vi "S4GUI.vi"(7 "Tab ObsEng":enum32{"Obs", "CCD modes", "Guider", "Eng"}(tab)) -> ()   [LabVIEW 2018] (continued)
                    n880 = Not(x=w1537) -> (.not. x?=w1558:bool)
                    n881 = Not(x=w1536) -> (.not. x?=w1557:bool)
                    n882 = Not(x=w1535) -> (.not. x?=w1559:bool)
                    n883 = property on="Acquisition Mode 2" class="Ring (strict)"("Blinking"=w1553) -> ()  [unwired: 2 in, 2 out]
                    n884 = property on="Readout Rate 2" class="Ring (strict)"("Blinking"=w1556) -> ()  [unwired: 2 in, 2 out]
                    n885 = property on="Vertical Shift Speed 2" class="Ring (strict)"("Blinking"=w1554) -> ()  [unwired: 2 in, 2 out]
                    n886 = property on="CCD EM Mode 2" class="Ring (strict)"("Blinking"=w1555) -> ()  [unwired: 2 in, 2 out]
                    n887 = property on="Trigger Mode 2" class="Ring (strict)"("Blinking"=w1558) -> ()  [unwired: 2 in, 2 out]
                    n888 = property on="Read Mode 2" class="Ring (strict)"("Blinking"=w1557) -> ()  [unwired: 2 in, 2 out]
                    n889 = property on="Pre-amplification Gain 2" class="Ring (strict)"("Blinking"=w1559) -> ()  [unwired: 2 in, 2 out]
                  }
                }
                n890 = local read "Cameras Cluster"() -> (w1523:T7)
                n891 = Bundle By Name(cluster=w1523, "Current Configuration.Image Initial Line 2"=w1486, "Current Configuration.Image Initial Column 2"=w1484, "Current Configuration.Image Final Line 2"=w1487, "Current Configuration.Image FInal Column 2"=w1485, "Current Configuration.Vertical Binning 2"=w1490, "Current Configuration.Horizontal Binning 2"=w1521, "Current Configuration.Pre-amplification Gain 2"=w1489, "Current Configuration.CCD EM Gain 2"=w1488, "Current Configuration.Readout Rate 2"=w1483, "Current Configuration.Shutter Openning Time 2"=w1520, "Current Configuration.Shutter Closing Time 2"=w1519, "Current Configuration.Vertical Shift Speed 2"=w1518, "Current Configuration.Read Mode 2"=w1517, "Current Configuration.Vertical Clock Voltage 2"=w1516, "Current Configuration.A/D Channel 2"=w1515, "Current Configuration.Shutter Mode 2"=w1512, "Current Configuration.Shutter TTL 2"=w1513, "Current Configuration.Trigger Mode 2"=w1491, "Current Configuration.Frame Transfer 2"=w1492, "Current Configuration.Acquisition Mode 2"=w1514, "Current Configuration.CCD EM Mode 2"=w1482) -> (w1522:T7)
                n892 = local write "PA2"(w1477) -> ()
                n893 = local write "B2"(w1476) -> ()
                n894 = local write "EA2"(w1478) -> ()
                n895 = local write "SI2"(w1473) -> ()
                n896 = local write "RO2"(w1474) -> ()
                n897 = local write "G2"(w1475) -> ()
                n898 = local write "Cameras Cluster"(w1522) -> ()
                n899 = Compound Arithmetic op=AND(w1497, w1496, w1495, w1494, w1470, w1469, w1493, w1504, w1503, w1502, w1501, w1500, w1499, w1498, w1511, w1510, w1509, w1508, w1507, w1506, w1505) -> (w1468:bool)
                "CCD checked 2" <- w1468
                n900 = disable-structure shown="Disabled" {
                  disable-tunnel: w1468 -> [w1525 _]
                  frame Disabled {
                    n901 = Select(t=u32 1244955, s=w1525, f=u32 16718848) -> (s? t:f=w1528:u32)
                    n902 = property on="CCD checked 2" class="Bool (strict)"("Caption.BG Color"=w1528) -> ()  [unwired: 2 in, 2 out]
                  }
                  frame Enabled {
                  }
                }
                n903 = property on="Acquisition Mode 2" class="Ring (strict)"("DisabledEnum"=w1471) -> ()  [unwired: 2 in, 2 out]
                n904 = property on="Readout Rate 2" class="Ring (strict)"("DisabledEnum"=w1471) -> ()  [unwired: 2 in, 2 out]
                n905 = property on="Vertical Shift Speed 2" class="Ring (strict)"("DisabledEnum"=w1471) -> ()  [unwired: 2 in, 2 out]
                n906 = property on="CCD EM Mode 2" class="Ring (strict)"("DisabledEnum"=w1471) -> ()  [unwired: 2 in, 2 out]
                n907 = property on="Shutter Openning Time 2" class="DigNum (strict)"("DisabledEnum"=w1471) -> ()  [unwired: 2 in, 2 out]
                n908 = property on="Shutter Closing Time 2" class="DigNum (strict)"("DisabledEnum"=w1471) -> ()  [unwired: 2 in, 2 out]
                n909 = property on="Vertical Binning 2" class="DigNum (strict)"("DisabledEnum"=w1471) -> ()  [unwired: 2 in, 2 out]
                n910 = property on="Horizontal Binning 2" class="DigNum (strict)"("DisabledEnum"=w1471) -> ()  [unwired: 2 in, 2 out]
                n911 = property on="Trigger Mode 2" class="Ring (strict)"("DisabledEnum"=w1471) -> ()  [unwired: 2 in, 2 out]
                n912 = property on="Read Mode 2" class="Ring (strict)"("DisabledEnum"=w1471) -> ()  [unwired: 2 in, 2 out]
                n913 = property on="Pre-amplification Gain 2" class="Ring (strict)"("DisabledEnum"=w1471) -> ()  [unwired: 2 in, 2 out]
                n914 = property on="CCD EM Gain 2" class="DigNum (strict)"("DisabledEnum"=w1471) -> ()  [unwired: 2 in, 2 out]
                n915 = property on="Shutter Mode 2" class="Ring (strict)"("DisabledEnum"=w1471) -> ()  [unwired: 2 in, 2 out]
                n916 = property on="Shutter TTL 2" class="Ring (strict)"("DisabledEnum"=w1471) -> ()  [unwired: 2 in, 2 out]
                n917 = property on="Image FInal Column 2" class="DigNum (strict)"("DisabledEnum"=w1471) -> ()  [unwired: 2 in, 2 out]
                n918 = property on="Frame Transfer 2" class="Bool (strict)"("DisabledEnum"=w1471) -> ()  [unwired: 2 in, 2 out]
                n919 = property on="Vertical Clock Voltage 2" class="Ring (strict)"("DisabledEnum"=w1471) -> ()  [unwired: 2 in, 2 out]
                n920 = property on="A/D Channel 2" class="DigNum (strict)"("DisabledEnum"=w1471) -> ()  [unwired: 2 in, 2 out]
                n921 = property on="Image Initial Line 2" class="DigNum (strict)"("DisabledEnum"=w1471) -> ()  [unwired: 2 in, 2 out]
                n922 = property on="Image Initial Column 2" class="DigNum (strict)"("DisabledEnum"=w1471) -> ()  [unwired: 2 in, 2 out]
                n923 = property on="Image Final Line 2" class="DigNum (strict)"("DisabledEnum"=w1471) -> ()  [unwired: 2 in, 2 out]
              }
              frame #17 {
                # "Carrega coluna do Channel 3"
                # "Aba:  Eng->Camera"
                n924 = Unbundle By Name(w1687) -> ("ChannelC_CCD"=w1657:T29, "CHC_Checked Params"=w1672:T14, "ChannelC_Status.connection"=w1650:bool)
                n925 = Unbundle By Name(w1672) -> ("ACQUISITION_MODE"=w1639:bool, "TRIGGER_MODE"=w1638:bool, "READ_MODE"=w1637:bool, "PREAMP"=w1636:bool, "READOUT_RATE"=w1635:bool, "VERTICAL_SHIFT_SPEED"=w1634:bool, "EM_MODE"=w1633:bool, "EM_GAIN"=w1670:bool, "SHUTTER_MODE"=w1669:bool, "SHUTTER_TTL"=w1668:bool, "SHUTTER_OPENING_TIME"=w1667:bool, "SHUTTER_CLOSING_TIME"=w1649:bool, "VBIN"=w1641:bool, "HBIN"=w1640:bool, "INITIAL_LINE"=w1648:bool, "INITIAL_COLUMN"=w1647:bool, "FINAL_LINE"=w1646:bool, "FINAL_COLUMN"=w1645:bool, "FRAME_TRANSFER"=w1644:bool, "VERTICAL_CLOCK_VOLTAGE"=w1643:bool, "AD_CHANNEL"=w1642:bool)
                n926 = case shown="True" w1650 {
                  tunnel: w1657 -> [_ w1740]
                  tunnel: [w1733 w1739] -> w1656
                  tunnel: [w1733 w1738] -> w1655
                  tunnel: [w1733 w1737] -> w1654
                  tunnel: [w1733 w1736] -> w1653
                  tunnel: [w1733 w1735] -> w1652
                  tunnel: [w1733 w1734] -> w1651
                  frame False {
                    w1733 = ""
                  }
                  frame True {
                    n927 = stacked-sequence "Atualizacao dos indicadores inferiores do CANAL C da tela principal" {
                      tunnel: w1740 -> [w1755 w1758 w1763 w1772 w1775 w1779]
                      tunnel: [w1741 _ _ _ _ _] -> w1739
                      tunnel: [_ w1756 _ _ _ _] -> w1738
                      tunnel: [_ _ w1761 _ _ _] -> w1737
                      tunnel: [_ _ _ w1766 _ _] -> w1736
                      tunnel: [_ _ _ _ w1773 _] -> w1735
                      tunnel: [_ _ _ _ _ w1776] -> w1734
                      frame #0 {
                        # "SubImage"
                        n928 = Unbundle By Name(w1755) -> ("INITIAL_LINE"=w1753:u16, "FINAL_LINE"=w1752:u16, "INITIAL_COLUMN"=w1751:u16, "FINAL_COLUMN"=w1750:u16)
                        n929 = Number To Decimal String(number=w1753) -> (decimal integer string=w1749:string)  [unwired: 1 in]
                        n930 = Number To Decimal String(number=w1752) -> (decimal integer string=w1747:string)  [unwired: 1 in]
                        n931 = Number To Decimal String(number=w1751) -> (decimal integer string=w1745:string)  [unwired: 1 in]
                        n932 = Number To Decimal String(number=w1750) -> (decimal integer string=w1743:string)  [unwired: 1 in]
                        n933 = Concatenate Strings("[", w1749, ":", w1747, ",", w1745, ":", w1743, "]") -> (w1741:string)
                      }
                      frame #1 {
                        # "Em Active"
                        n934 = Unbundle By Name(w1758) -> ("EM_MODE"=w1757:u8)
                        n935 = case shown="0, Default" w1757 {
                          tunnel: ["Electron M." ("EmActive1") "Convent." ("EmActive1")] -> w1756
                          frame 0, Default {
                          }
                          frame 1 {
                          }
                        }
                      }
                      frame #2 {
                        # "Pre Amp"
                        n936 = Unbundle By Name(w1763) -> ("PREAMP"=w1762:u8)
                        n937 = case shown="1" w1762 {
                          tunnel: ["Gain 1" ("EmActive1") "Gain 2" ("EmActive1")] -> w1761
                          frame 0, Default {
                          }
                          frame 1 {
                          }
                        }
                      }
                      frame #3 {
                        # "Binning"
                        n938 = Unbundle By Name(w1772) -> ("VBIN"=w1771:u16, "HBIN"=w1770:u16)
                        n939 = Number To Decimal String(number=w1770) -> (decimal integer string=w1767:string)  [unwired: 1 in]
                        n940 = Number To Decimal String(number=w1771) -> (decimal integer string=w1769:string)  [unwired: 1 in]
                        n941 = Concatenate Strings(w1769, "x", w1767) -> (w1766:string)
                      }
                      frame #4 {
                        # "Gain"
                        n942 = Unbundle By Name(w1775) -> ("EM_GAIN"=w1774:u16)
                        n943 = Number To Decimal String(number=w1774) -> (decimal integer string=w1773:string)  [unwired: 1 in]
                      }
                      frame #5 {
                        # "Readout"
                        n944 = Unbundle By Name(w1779) -> ("EM_MODE"=w1778:u8, "READOUT_RATE"=w1777:u8)
                        n945 = case shown="0, Default" w1778 {
                          tunnel: w1777 -> [w1781 w1787]
                          tunnel: [w1780 w1786] -> w1776
                          frame 0, Default {
                            n946 = case shown="3" w1781 {
                              tunnel: ["30 MHz" ("EmActive1") "20 MHz" ("EmActive1") "10 MHz" ("EmActive1") "1 MHz" ("EmActive1")] -> w1780
                              frame 0, Default {
                              }
                              frame 1 {
                              }
                              frame 2 {
                              }
                              frame 3 {
                              }
                            }
                          }
                          frame 1 {
                            n947 = case shown="1" w1787 {
                              tunnel: ["1 MHz" ("EmActive1") "0.1 MHz" ("EmActive1")] -> w1786
                              frame 0, Default {
                              }
                              frame 1 {
                              }
                            }
                          }
                        }
                      }
                    }
                  }
                }
                n948 = Unbundle By Name(w1657) -> ("INITIAL_LINE"=w1662:u16, "INITIAL_COLUMN"=w1660:u16, "FINAL_LINE"=w1663:u16, "FINAL_COLUMN"=w1661:u16, "VBIN"=w1666:u16, "HBIN"=w1684:u16, "PREAMP"=w1665:u8, "EM_GAIN"=w1664:u16, "READOUT_RATE"=w1659:u8, "SHUTTER_OPENNING_TIME"=w1683:u16, "SHUTTER_CLOSING_TIME"=w1682:u16, "VERTICAL_SHIFT_SPEED"=w1681:u8, "READ_MODE"=w1680:u8, "VERTICAL_CLOCK_VOLTAGE"=w1679:u8, "AD_CHANNEL"=w1678:u32, "SHUTTER_MODE"=w1673:u8, "SHUTTER_TTL"=w1674:u8, "TRIGGER_MODE"=w1675:u8, "FRAME_TRANSFER"=w1676:bool, "ACQUISITION_MODE"=w1677:u8, "EM_MODE"=w1658:u8)
                n949 = local read "CH3 on"() -> (w1632:bool)
                n950 = case shown="True" w1632 {
                  tunnel: w1670 -> [_ w1713]
                  tunnel: w1669 -> [_ w1712]
                  tunnel: w1668 -> [_ w1710]
                  tunnel: w1667 -> [_ w1709]
                  tunnel: w1649 -> [_ w1708]
                  tunnel: w1648 -> [_ w1707]
                  tunnel: w1647 -> [_ w1706]
                  tunnel: w1646 -> [_ w1705]
                  tunnel: w1645 -> [_ w1704]
                  tunnel: w1644 -> [_ w1703]
                  tunnel: w1643 -> [_ w1702]
                  tunnel: w1642 -> [_ w1701]
                  tunnel: w1641 -> [_ w1700]
                  tunnel: w1640 -> [_ w1699]
                  tunnel: w1639 -> [_ w1698]
                  tunnel: w1638 -> [_ w1697]
                  tunnel: w1637 -> [_ w1696]
                  tunnel: w1636 -> [_ w1695]
                  tunnel: w1635 -> [_ w1694]
                  tunnel: w1634 -> [_ w1693]
                  tunnel: w1633 -> [_ w1692]
                  tunnel: [T12."Disabled and Grayed Out" ("Disabled") T12."Enabled" ("Disabled")] -> w1631
                  frame False {
                    w1688 = FALSE
                    n951 = property on="Image Initial Line 3" class="DigNum (strict)"("Blinking"=w1688) -> ()  [unwired: 2 in, 2 out]
                    n952 = property on="Image Initial Column 3" class="DigNum (strict)"("Blinking"=w1688) -> ()  [unwired: 2 in, 2 out]
                    n953 = property on="Image Final Line 3" class="DigNum (strict)"("Blinking"=w1688) -> ()  [unwired: 2 in, 2 out]
                    n954 = property on="Image FInal Column 3" class="DigNum (strict)"("Blinking"=w1688) -> ()  [unwired: 2 in, 2 out]
                    n955 = property on="Frame Transfer 3" class="Bool (strict)"("Blinking"=w1688) -> ()  [unwired: 2 in, 2 out]
                    n956 = property on="Vertical Clock Voltage 3" class="Ring (strict)"("Blinking"=w1688) -> ()  [unwired: 2 in, 2 out]
                    n957 = property on="A/D Channel 3" class="DigNum (strict)"("Blinking"=w1688) -> ()  [unwired: 2 in, 2 out]
                    n958 = property on="CCD EM Gain 3" class="DigNum (strict)"("Blinking"=w1688) -> ()  [unwired: 2 in, 2 out]
                    n959 = property on="Shutter Mode 3" class="Ring (strict)"("Blinking"=w1688) -> ()  [unwired: 2 in, 2 out]
                    n960 = property on="Shutter TTL 3" class="Ring (strict)"("Blinking"=w1688) -> ()  [unwired: 2 in, 2 out]
                    n961 = property on="Shutter Openning Time 3" class="DigNum (strict)"("Blinking"=w1688) -> ()  [unwired: 2 in, 2 out]
                    n962 = property on="Shutter Closing Time 3" class="DigNum (strict)"("Blinking"=w1688) -> ()  [unwired: 2 in, 2 out]
                    n963 = property on="Vertical Binning 3" class="DigNum (strict)"("Blinking"=w1688) -> ()  [unwired: 2 in, 2 out]
                    n964 = property on="Horizontal Binning 3" class="DigNum (strict)"("Blinking"=w1688) -> ()  [unwired: 2 in, 2 out]
                    n965 = property on="Acquisition Mode 3" class="Ring (strict)"("Blinking"=w1688) -> ()  [unwired: 2 in, 2 out]
                    n966 = property on="Vertical Shift Speed 3" class="Ring (strict)"("Blinking"=w1688) -> ()  [unwired: 2 in, 2 out]
                    n967 = property on="Trigger Mode 3" class="Ring (strict)"("Blinking"=w1688) -> ()  [unwired: 2 in, 2 out]
                    n968 = property on="Read Mode 3" class="Ring (strict)"("Blinking"=w1688) -> ()  [unwired: 2 in, 2 out]
                    n969 = property on="Readout Rate 3" class="Ring (strict)"("Blinking"=w1688) -> ()  [unwired: 2 in, 2 out]
                    n970 = property on="CCD EM Mode 3" class="Ring (strict)"("Blinking"=w1688) -> ()  [unwired: 2 in, 2 out]
                    n971 = property on="Pre-amplification Gain 3" class="Ring (strict)"("Blinking"=w1688) -> ()  [unwired: 2 in, 2 out]
                  }
                  frame True {
                    n972 = Not(x=w1707) -> (.not. x?=w1690:bool)
                    n973 = Not(x=w1706) -> (.not. x?=w1731:bool)
                    n974 = Not(x=w1705) -> (.not. x?=w1732:bool)
                    n975 = Not(x=w1704) -> (.not. x?=w1730:bool)
                    n976 = Not(x=w1703) -> (.not. x?=w1728:bool)
                    n977 = Not(x=w1702) -> (.not. x?=w1729:bool)
                    n978 = Not(x=w1701) -> (.not. x?=w1727:bool)
                    n979 = property on="Image FInal Column 3" class="DigNum (strict)"("Blinking"=w1730) -> ()  [unwired: 2 in, 2 out]
                    n980 = property on="Frame Transfer 3" class="Bool (strict)"("Blinking"=w1728) -> ()  [unwired: 2 in, 2 out]
                    n981 = property on="Vertical Clock Voltage 3" class="Ring (strict)"("Blinking"=w1729) -> ()  [unwired: 2 in, 2 out]
                    n982 = property on="Image Initial Line 3" class="DigNum (strict)"("Blinking"=w1690) -> ()  [unwired: 2 in, 2 out]
                    n983 = property on="Image Initial Column 3" class="DigNum (strict)"("Blinking"=w1731) -> ()  [unwired: 2 in, 2 out]
                    n984 = property on="Image Final Line 3" class="DigNum (strict)"("Blinking"=w1732) -> ()  [unwired: 2 in, 2 out]
                    n985 = property on="A/D Channel 3" class="DigNum (strict)"("Blinking"=w1727) -> ()  [unwired: 2 in, 2 out]
                    n986 = Not(x=w1709) -> (.not. x?=w1723:bool)
                    n987 = Not(x=w1708) -> (.not. x?=w1725:bool)
                    n988 = Not(x=w1700) -> (.not. x?=w1724:bool)
                    n989 = Not(x=w1699) -> (.not. x?=w1726:bool)
                    n990 = Not(x=w1713) -> (.not. x?=w1722:bool)
                    n991 = Not(x=w1712) -> (.not. x?=w1711:bool)
                    n992 = Not(x=w1710) -> (.not. x?=w1721:bool)
                    n993 = property on="Shutter Openning Time 3" class="DigNum (strict)"("Blinking"=w1723) -> ()  [unwired: 2 in, 2 out]
                    n994 = property on="Shutter Closing Time 3" class="DigNum (strict)"("Blinking"=w1725) -> ()  [unwired: 2 in, 2 out]
                    n995 = property on="Vertical Binning 3" class="DigNum (strict)"("Blinking"=w1724) -> ()  [unwired: 2 in, 2 out]
                    n996 = property on="Horizontal Binning 3" class="DigNum (strict)"("Blinking"=w1726) -> ()  [unwired: 2 in, 2 out]
                    n997 = property on="CCD EM Gain 3" class="DigNum (strict)"("Blinking"=w1722) -> ()  [unwired: 2 in, 2 out]
                    n998 = property on="Shutter Mode 3" class="Ring (strict)"("Blinking"=w1711) -> ()  [unwired: 2 in, 2 out]
                    n999 = property on="Shutter TTL 3" class="Ring (strict)"("Blinking"=w1721) -> ()  [unwired: 2 in, 2 out]
                    n1000 = Not(x=w1698) -> (.not. x?=w1714:bool)
                    n1001 = Not(x=w1694) -> (.not. x?=w1717:bool)
                    n1002 = Not(x=w1693) -> (.not. x?=w1715:bool)
                    n1003 = Not(x=w1692) -> (.not. x?=w1716:bool)
                    n1004 = Not(x=w1697) -> (.not. x?=w1719:bool)
                    n1005 = Not(x=w1696) -> (.not. x?=w1718:bool)
                    n1006 = Not(x=w1695) -> (.not. x?=w1720:bool)
                    n1007 = property on="Acquisition Mode 3" class="Ring (strict)"("Blinking"=w1714) -> ()  [unwired: 2 in, 2 out]
                    n1008 = property on="Readout Rate 3" class="Ring (strict)"("Blinking"=w1717) -> ()  [unwired: 2 in, 2 out]
                    n1009 = property on="Vertical Shift Speed 3" class="Ring (strict)"("Blinking"=w1715) -> ()  [unwired: 2 in, 2 out]
                    n1010 = property on="CCD EM Mode 3" class="Ring (strict)"("Blinking"=w1716) -> ()  [unwired: 2 in, 2 out]
                    n1011 = property on="Trigger Mode 3" class="Ring (strict)"("Blinking"=w1719) -> ()  [unwired: 2 in, 2 out]
                    n1012 = property on="Read Mode 3" class="Ring (strict)"("Blinking"=w1718) -> ()  [unwired: 2 in, 2 out]
                    n1013 = property on="Pre-amplification Gain 3" class="Ring (strict)"("Blinking"=w1720) -> ()  [unwired: 2 in, 2 out]
                  }
                }
                n1014 = local write "RO3"(w1651) -> ()
                n1015 = local write "B3"(w1653) -> ()
                n1016 = local write "PA3"(w1654) -> ()
                n1017 = local write "EA3"(w1655) -> ()
                n1018 = local write "G3"(w1652) -> ()
                n1019 = local write "SI3"(w1656) -> ()
                n1020 = local read "Cameras Cluster"() -> (w1686:T7)
                n1021 = Bundle By Name(cluster=w1686, "Current Configuration.Image Initial Line 3"=w1662, "Current Configuration.Image Initial Column 3"=w1660, "Current Configuration.Image Final Line 3"=w1663, "Current Configuration.Image FInal Column 3"=w1661, "Current Configuration.Vertical Binning 3"=w1666, "Current Configuration.Horizontal Binning 3"=w1684, "Current Configuration.Pre-amplification Gain 3"=w1665, "Current Configuration.CCD EM Gain 3"=w1664, "Current Configuration.Readout Rate 3"=w1659, "Current Configuration.Shutter Openning Time 3"=w1683, "Current Configuration.Shutter Closing Time 3"=w1682, "Current Configuration.Vertical Shift Speed 3"=w1681, "Current Configuration.Read Mode 3"=w1680, "Current Configuration.Vertical Clock Voltage 3"=w1679, "Current Configuration.A/D Channel 3"=w1678, "Current Configuration.Shutter Mode 3"=w1673, "Current Configuration.Shutter TTL 3"=w1674, "Current Configuration.Trigger Mode 3"=w1675, "Current Configuration.Frame Transfer 3"=w1676, "Current Configuration.Acquisition Mode 3"=w1677, "Current Configuration.CCD EM Mode 3"=w1658) -> (w1685:T7)
                n1022 = local write "Cameras Cluster"(w1685) -> ()
                n1023 = Compound Arithmetic op=AND(w1639, w1638, w1637, w1636, w1635, w1634, w1633, w1670, w1669, w1668, w1667, w1649, w1641, w1640, w1648, w1647, w1646, w1645, w1644, w1643, w1642) -> (→"CCD checked 3":bool)
                n1024 = property on="Image Initial Line 3" class="DigNum (strict)"("DisabledEnum"=w1631) -> ()  [unwired: 2 in, 2 out]
                n1025 = property on="Image Initial Column 3" class="DigNum (strict)"("DisabledEnum"=w1631) -> ()  [unwired: 2 in, 2 out]
                n1026 = property on="Image Final Line 3" class="DigNum (strict)"("DisabledEnum"=w1631) -> ()  [unwired: 2 in, 2 out]
                n1027 = property on="Image FInal Column 3" class="DigNum (strict)"("DisabledEnum"=w1631) -> ()  [unwired: 2 in, 2 out]
                n1028 = property on="Frame Transfer 3" class="Bool (strict)"("DisabledEnum"=w1631) -> ()  [unwired: 2 in, 2 out]
                n1029 = property on="Horizontal Binning 3" class="DigNum (strict)"("DisabledEnum"=w1631) -> ()  [unwired: 2 in, 2 out]
                n1030 = property on="Vertical Clock Voltage 3" class="Ring (strict)"("DisabledEnum"=w1631) -> ()  [unwired: 2 in, 2 out]
                n1031 = property on="CCD EM Gain 3" class="DigNum (strict)"("DisabledEnum"=w1631) -> ()  [unwired: 2 in, 2 out]
                n1032 = property on="Shutter Mode 3" class="Ring (strict)"("DisabledEnum"=w1631) -> ()  [unwired: 2 in, 2 out]
                n1033 = property on="Shutter Openning Time 3" class="DigNum (strict)"("DisabledEnum"=w1631) -> ()  [unwired: 2 in, 2 out]
                n1034 = property on="Shutter Closing Time 3" class="DigNum (strict)"("DisabledEnum"=w1631) -> ()  [unwired: 2 in, 2 out]
                n1035 = property on="Vertical Binning 3" class="DigNum (strict)"("DisabledEnum"=w1631) -> ()  [unwired: 2 in, 2 out]
                n1036 = property on="Shutter TTL 3" class="Ring (strict)"("DisabledEnum"=w1631) -> ()  [unwired: 2 in, 2 out]
                n1037 = property on="Pre-amplification Gain 3" class="Ring (strict)"("DisabledEnum"=w1631) -> ()  [unwired: 2 in, 2 out]
                n1038 = property on="Acquisition Mode 3" class="Ring (strict)"("DisabledEnum"=w1631) -> ()  [unwired: 2 in, 2 out]
                n1039 = property on="Trigger Mode 3" class="Ring (strict)"("DisabledEnum"=w1631) -> ()  [unwired: 2 in, 2 out]
                n1040 = property on="Read Mode 3" class="Ring (strict)"("DisabledEnum"=w1631) -> ()  [unwired: 2 in, 2 out]
                n1041 = property on="Readout Rate 3" class="Ring (strict)"("DisabledEnum"=w1631) -> ()  [unwired: 2 in, 2 out]
                n1042 = property on="A/D Channel 3" class="DigNum (strict)"("DisabledEnum"=w1631) -> ()  [unwired: 2 in, 2 out]
                n1043 = property on="Vertical Shift Speed 3" class="Ring (strict)"("DisabledEnum"=w1631) -> ()  [unwired: 2 in, 2 out]
                n1044 = property on="CCD EM Mode 3" class="Ring (strict)"("DisabledEnum"=w1631) -> ()  [unwired: 2 in, 2 out]
              }
              frame #18 {
                # "Carrega coluna do Channel 4"
                # "Aba:  Eng->Camera"
                n1045 = Unbundle By Name(w1846) -> ("ChannelD_CCD"=w1799:T29, "CHD_Checked Params"=w1831:T14, "ChannelD_Status.connection"=w1798:bool)
                n1046 = Unbundle By Name(w1831) -> ("ACQUISITION_MODE"=w1815:bool, "TRIGGER_MODE"=w1814:bool, "READ_MODE"=w1813:bool, "PREAMP"=w1812:bool, "READOUT_RATE"=w1811:bool, "VERTICAL_SHIFT_SPEED"=w1810:bool, "EM_MODE"=w1809:bool, "EM_GAIN"=w1822:bool, "SHUTTER_MODE"=w1821:bool, "SHUTTER_TTL"=w1820:bool, "SHUTTER_OPENING_TIME"=w1819:bool, "SHUTTER_CLOSING_TIME"=w1818:bool, "VBIN"=w1817:bool, "HBIN"=w1816:bool, "INITIAL_LINE"=w1829:bool, "INITIAL_COLUMN"=w1828:bool, "FINAL_LINE"=w1827:bool, "FINAL_COLUMN"=w1826:bool, "FRAME_TRANSFER"=w1825:bool, "VERTICAL_CLOCK_VOLTAGE"=w1824:bool, "AD_CHANNEL"=w1823:bool)
                n1047 = case shown="True" w1798 {
                  tunnel: w1799 -> [_ w1899]
                  tunnel: [w1892 w1898] -> w1797
                  tunnel: [w1892 w1897] -> w1796
                  tunnel: [w1892 w1896] -> w1795
                  tunnel: [w1892 w1895] -> w1794
                  tunnel: [w1892 w1894] -> w1793
                  tunnel: [w1892 w1893] -> w1792
                  frame False {
                    w1892 = ""
                  }
                  frame True {
                    n1048 = stacked-sequence "Atualizacao dos indicadores inferiores do CANAL D da tela principal" {
                      tunnel: w1899 -> [w1914 w1917 w1922 w1931 w1934 w1938]
                      tunnel: [w1900 _ _ _ _ _] -> w1898
                      tunnel: [_ w1915 _ _ _ _] -> w1897
                      tunnel: [_ _ w1920 _ _ _] -> w1896
                      tunnel: [_ _ _ w1925 _ _] -> w1895
                      tunnel: [_ _ _ _ w1932 _] -> w1894
                      tunnel: [_ _ _ _ _ w1935] -> w1893
                      frame #0 {
                        # "SubImage"
                        n1049 = Unbundle By Name(w1914) -> ("INITIAL_LINE"=w1912:u16, "FINAL_LINE"=w1911:u16, "INITIAL_COLUMN"=w1910:u16, "FINAL_COLUMN"=w1909:u16)
                        n1050 = Number To Decimal String(number=w1912) -> (decimal integer string=w1908:string)  [unwired: 1 in]
                        n1051 = Number To Decimal String(number=w1911) -> (decimal integer string=w1906:string)  [unwired: 1 in]
                        n1052 = Number To Decimal String(number=w1910) -> (decimal integer string=w1904:string)  [unwired: 1 in]
                        n1053 = Number To Decimal String(number=w1909) -> (decimal integer string=w1902:string)  [unwired: 1 in]
                        n1054 = Concatenate Strings("[", w1908, ":", w1906, ",", w1904, ":", w1902, "]") -> (w1900:string)
                      }
                      frame #1 {
                        # "Em Active"
                        n1055 = Unbundle By Name(w1917) -> ("EM_MODE"=w1916:u8)
                        n1056 = case shown="0, Default" w1916 {
                          tunnel: ["Electron M." ("EmActive1") "Convent." ("EmActive1")] -> w1915
                          frame 0, Default {
                          }
                          frame 1 {
                          }
                        }
                      }
                      frame #2 {
                        # "Pre Amp"
                        n1057 = Unbundle By Name(w1922) -> ("PREAMP"=w1921:u8)
                        n1058 = case shown="1" w1921 {
                          tunnel: ["Gain 1" ("EmActive1") "Gain 2" ("EmActive1")] -> w1920
                          frame 0, Default {
                          }
                          frame 1 {
                          }
                        }
                      }
                      frame #3 {
                        # "Binning"
                        n1059 = Unbundle By Name(w1931) -> ("VBIN"=w1930:u16, "HBIN"=w1929:u16)
                        n1060 = Number To Decimal String(number=w1929) -> (decimal integer string=w1926:string)  [unwired: 1 in]
                        n1061 = Number To Decimal String(number=w1930) -> (decimal integer string=w1928:string)  [unwired: 1 in]
                        n1062 = Concatenate Strings(w1928, "x", w1926) -> (w1925:string)
                      }
                      frame #4 {
                        # "Gain"
                        n1063 = Unbundle By Name(w1934) -> ("EM_GAIN"=w1933:u16)
                        n1064 = Number To Decimal String(number=w1933) -> (decimal integer string=w1932:string)  [unwired: 1 in]
                      }
                      frame #5 {
                        # "Readout"
                        n1065 = Unbundle By Name(w1938) -> ("EM_MODE"=w1937:u8, "READOUT_RATE"=w1936:u8)
                        n1066 = case shown="0, Default" w1937 {
                          tunnel: w1936 -> [w1940 w1946]
                          tunnel: [w1939 w1945] -> w1935
                          frame 0, Default {
                            n1067 = case shown="3" w1940 {
                              tunnel: ["30 MHz" ("EmActive1") "20 MHz" ("EmActive1") "10 MHz" ("EmActive1") "1 MHz" ("EmActive1")] -> w1939
                              frame 0, Default {
                              }
                              frame 1 {
                              }
                              frame 2 {
                              }
                              frame 3 {
                              }
                            }
                          }
                          frame 1 {
                            n1068 = case shown="0, Default" w1946 {
                              tunnel: ["1 MHz" ("EmActive1") "0.1 MHz" ("EmActive1")] -> w1945
                              frame 0, Default {
                              }
                              frame 1 {
                              }
                            }
                          }
                        }
                      }
                    }
                  }
                }
                n1069 = Unbundle By Name(w1799) -> ("INITIAL_LINE"=w1804:u16, "INITIAL_COLUMN"=w1802:u16, "FINAL_LINE"=w1805:u16, "FINAL_COLUMN"=w1803:u16, "VBIN"=w1808:u16, "HBIN"=w1843:u16, "PREAMP"=w1807:u8, "EM_GAIN"=w1806:u16, "READOUT_RATE"=w1801:u8, "SHUTTER_OPENNING_TIME"=w1842:u16, "SHUTTER_CLOSING_TIME"=w1841:u16, "VERTICAL_SHIFT_SPEED"=w1840:u8, "READ_MODE"=w1839:u8, "VERTICAL_CLOCK_VOLTAGE"=w1838:u8, "AD_CHANNEL"=w1837:u32, "SHUTTER_MODE"=w1832:u8, "SHUTTER_TTL"=w1833:u8, "TRIGGER_MODE"=w1834:u8, "FRAME_TRANSFER"=w1835:bool, "ACQUISITION_MODE"=w1836:u8, "EM_MODE"=w1800:u8)
                n1070 = local read "CH4 on"() -> (w1791:bool)
                n1071 = case shown="False" w1791 {
                  tunnel: w1829 -> [_ w1871]
                  tunnel: w1828 -> [_ w1870]
                  tunnel: w1827 -> [_ w1869]
                  tunnel: w1826 -> [_ w1868]
                  tunnel: w1825 -> [_ w1867]
                  tunnel: w1824 -> [_ w1866]
                  tunnel: w1823 -> [_ w1865]
                  tunnel: w1822 -> [_ w1864]
                  tunnel: w1821 -> [_ w1863]
                  tunnel: w1820 -> [_ w1862]
                  tunnel: w1819 -> [_ w1861]
                  tunnel: w1818 -> [_ w1860]
                  tunnel: w1817 -> [_ w1859]
                  tunnel: w1816 -> [_ w1858]
                  tunnel: w1815 -> [_ w1857]
                  tunnel: w1814 -> [_ w1856]
                  tunnel: w1813 -> [_ w1855]
                  tunnel: w1812 -> [_ w1853]
                  tunnel: w1811 -> [_ w1852]
                  tunnel: w1810 -> [_ w1851]
                  tunnel: w1809 -> [_ w1850]
                  tunnel: [T12."Disabled and Grayed Out" ("Disabled") T12."Enabled" ("Disabled")] -> w1790
                  frame False {
                    w1848 = FALSE ("Blinking")
                    n1072 = property on="Image FInal Column 4" class="DigNum (strict)"("Blinking"=w1848) -> ()  [unwired: 2 in, 2 out]
                    n1073 = property on="Frame Transfer 4" class="Bool (strict)"("Blinking"=w1848) -> ()  [unwired: 2 in, 2 out]
                    n1074 = property on="Vertical Clock Voltage 4" class="Ring (strict)"("Blinking"=w1848) -> ()  [unwired: 2 in, 2 out]
                    n1075 = property on="A/D Channel 4" class="DigNum (strict)"("Blinking"=w1848) -> ()  [unwired: 2 in, 2 out]
                    n1076 = property on="Image Initial Line 4" class="DigNum (strict)"("Blinking"=w1848) -> ()  [unwired: 2 in, 2 out]
                    n1077 = property on="Image Initial Column 4" class="DigNum (strict)"("Blinking"=w1848) -> ()  [unwired: 2 in, 2 out]
                    n1078 = property on="Image Final Line 4" class="DigNum (strict)"("Blinking"=w1848) -> ()  [unwired: 2 in, 2 out]
                    n1079 = property on="Shutter Openning Time 4" class="DigNum (strict)"("Blinking"=w1848) -> ()  [unwired: 2 in, 2 out]
                    n1080 = property on="Shutter Closing Time 4" class="DigNum (strict)"("Blinking"=w1848) -> ()  [unwired: 2 in, 2 out]
                    n1081 = property on="Vertical Binning 4" class="DigNum (strict)"("Blinking"=w1848) -> ()  [unwired: 2 in, 2 out]
                    n1082 = property on="Horizontal Binning 4" class="DigNum (strict)"("Blinking"=w1848) -> ()  [unwired: 2 in, 2 out]
                    n1083 = property on="CCD EM Gain 4" class="DigNum (strict)"("Blinking"=w1848) -> ()  [unwired: 2 in, 2 out]
                    n1084 = property on="Shutter Mode 4" class="Ring (strict)"("Blinking"=w1848) -> ()  [unwired: 2 in, 2 out]
                    n1085 = property on="Shutter TTL 4" class="Ring (strict)"("Blinking"=w1848) -> ()  [unwired: 2 in, 2 out]
                    n1086 = property on="Acquisition Mode 4" class="Ring (strict)"("Blinking"=w1848) -> ()  [unwired: 2 in, 2 out]
                    n1087 = property on="Readout Rate 4" class="Ring (strict)"("Blinking"=w1848) -> ()  [unwired: 2 in, 2 out]
                    n1088 = property on="Vertical Shift Speed 4" class="Ring (strict)"("Blinking"=w1848) -> ()  [unwired: 2 in, 2 out]
                    n1089 = property on="CCD EM Mode 4" class="Ring (strict)"("Blinking"=w1848) -> ()  [unwired: 2 in, 2 out]
                    n1090 = property on="Trigger Mode 4" class="Ring (strict)"("Blinking"=w1848) -> ()  [unwired: 2 in, 2 out]
                    n1091 = property on="Read Mode 4" class="Ring (strict)"("Blinking"=w1848) -> ()  [unwired: 2 in, 2 out]
                    n1092 = property on="Pre-amplification Gain 4" class="Ring (strict)"("Blinking"=w1848) -> ()  [unwired: 2 in, 2 out]
                  }
                  frame True {
                    n1093 = Not(x=w1868) -> (.not. x?=w1888:bool)
                    n1094 = Not(x=w1867) -> (.not. x?=w1886:bool)
                    n1095 = Not(x=w1866) -> (.not. x?=w1887:bool)
                    n1096 = Not(x=w1865) -> (.not. x?=w1885:bool)
                    n1097 = Not(x=w1871) -> (.not. x?=w1890:bool)
                    n1098 = Not(x=w1870) -> (.not. x?=w1889:bool)
                    n1099 = Not(x=w1869) -> (.not. x?=w1891:bool)
                    n1100 = property on="Image FInal Column 4" class="DigNum (strict)"("Blinking"=w1888) -> ()  [unwired: 2 in, 2 out]
                    n1101 = property on="Frame Transfer 4" class="Bool (strict)"("Blinking"=w1886) -> ()  [unwired: 2 in, 2 out]
                    n1102 = property on="Vertical Clock Voltage 4" class="Ring (strict)"("Blinking"=w1887) -> ()  [unwired: 2 in, 2 out]
                    n1103 = property on="A/D Channel 4" class="DigNum (strict)"("Blinking"=w1885) -> ()  [unwired: 2 in, 2 out]
                    n1104 = property on="Image Initial Line 4" class="DigNum (strict)"("Blinking"=w1890) -> ()  [unwired: 2 in, 2 out]
                    n1105 = property on="Image Initial Column 4" class="DigNum (strict)"("Blinking"=w1889) -> ()  [unwired: 2 in, 2 out]
                    n1106 = property on="Image Final Line 4" class="DigNum (strict)"("Blinking"=w1891) -> ()  [unwired: 2 in, 2 out]
                    n1107 = Not(x=w1861) -> (.not. x?=w1881:bool)
                    n1108 = Not(x=w1860) -> (.not. x?=w1883:bool)
                    n1109 = Not(x=w1859) -> (.not. x?=w1882:bool)
                    n1110 = Not(x=w1858) -> (.not. x?=w1884:bool)
                    n1111 = Not(x=w1864) -> (.not. x?=w1879:bool)
                    n1112 = Not(x=w1863) -> (.not. x?=w1880:bool)
                    n1113 = Not(x=w1862) -> (.not. x?=w1878:bool)
                    n1114 = property on="Shutter Openning Time 4" class="DigNum (strict)"("Blinking"=w1881) -> ()  [unwired: 2 in, 2 out]
                    n1115 = property on="Shutter Closing Time 4" class="DigNum (strict)"("Blinking"=w1883) -> ()  [unwired: 2 in, 2 out]
                    n1116 = property on="Vertical Binning 4" class="DigNum (strict)"("Blinking"=w1882) -> ()  [unwired: 2 in, 2 out]
                    n1117 = property on="Horizontal Binning 4" class="DigNum (strict)"("Blinking"=w1884) -> ()  [unwired: 2 in, 2 out]
                    n1118 = property on="CCD EM Gain 4" class="DigNum (strict)"("Blinking"=w1879) -> ()  [unwired: 2 in, 2 out]
                    n1119 = property on="Shutter Mode 4" class="Ring (strict)"("Blinking"=w1880) -> ()  [unwired: 2 in, 2 out]
                    n1120 = property on="Shutter TTL 4" class="Ring (strict)"("Blinking"=w1878) -> ()  [unwired: 2 in, 2 out]
                    n1121 = Not(x=w1857) -> (.not. x?=w1872:bool)
                    n1122 = Not(x=w1852) -> (.not. x?=w1875:bool)
                    n1123 = Not(x=w1851) -> (.not. x?=w1873:bool)
                    n1124 = Not(x=w1850) -> (.not. x?=w1874:bool)
                    n1125 = Not(x=w1856) -> (.not. x?=w1876:bool)
                    n1126 = Not(x=w1855) -> (.not. x?=w1854:bool)
                    n1127 = Not(x=w1853) -> (.not. x?=w1877:bool)
                    n1128 = property on="Acquisition Mode 4" class="Ring (strict)"("Blinking"=w1872) -> ()  [unwired: 2 in, 2 out]
                    n1129 = property on="Readout Rate 4" class="Ring (strict)"("Blinking"=w1875) -> ()  [unwired: 2 in, 2 out]
                    n1130 = property on="Vertical Shift Speed 4" class="Ring (strict)"("Blinking"=w1873) -> ()  [unwired: 2 in, 2 out]
                    n1131 = property on="CCD EM Mode 4" class="Ring (strict)"("Blinking"=w1874) -> ()  [unwired: 2 in, 2 out]
                    n1132 = property on="Trigger Mode 4" class="Ring (strict)"("Blinking"=w1876) -> ()  [unwired: 2 in, 2 out]
                    n1133 = property on="Read Mode 4" class="Ring (strict)"("Blinking"=w1854) -> ()  [unwired: 2 in, 2 out]
                    n1134 = property on="Pre-amplification Gain 4" class="Ring (strict)"("Blinking"=w1877) -> ()  [unwired: 2 in, 2 out]
                  }
                }
                n1135 = local write "SI4"(w1797) -> ()
                n1136 = local write "RO4"(w1792) -> ()
                n1137 = local write "PA4"(w1795) -> ()
                n1138 = local write "EA4"(w1796) -> ()
                n1139 = local write "G4"(w1793) -> ()
                n1140 = local write "B4"(w1794) -> ()
                n1141 = local read "Cameras Cluster"() -> (w1845:T7)
                n1142 = Bundle By Name(cluster=w1845, "Current Configuration.Image Initial Line 4"=w1804, "Current Configuration.Image Initial Column 4"=w1802, "Current Configuration.Image Final Line 4"=w1805, "Current Configuration.Image FInal Column 4"=w1803, "Current Configuration.Vertical Binning 4"=w1808, "Current Configuration.Horizontal Binning 4"=w1843, "Current Configuration.Pre-amplification Gain 4"=w1807, "Current Configuration.CCD EM Gain 4"=w1806, "Current Configuration.Readout Rate 4"=w1801, "Current Configuration.Shutter Openning Time 4"=w1842, "Current Configuration.Shutter Closing Time 4"=w1841, "Current Configuration.Vertical Shift Speed 4"=w1840, "Current Configuration.Read Mode 4"=w1839, "Current Configuration.Vertical Clock Voltage 4"=w1838, "Current Configuration.A/D Channel 4"=w1837, "Current Configuration.Shutter Mode 4"=w1832, "Current Configuration.Shutter TTL 4"=w1833, "Current Configuration.Trigger Mode 4"=w1834, "Current Configuration.Frame Transfer 4"=w1835, "Current Configuration.Acquisition Mode 4"=w1836, "Current Configuration.CCD EM Mode 4"=w1800) -> (w1844:T7)
                n1143 = local write "Cameras Cluster"(w1844) -> ()
                n1144 = Compound Arithmetic op=AND(w1815, w1814, w1813, w1812, w1811, w1810, w1809, w1822, w1821, w1820, w1819, w1818, w1817, w1816, w1829, w1828, w1827, w1826, w1825, w1824, w1823) -> (→"CCD checked 4":bool)
                n1145 = property on="Image FInal Column 4" class="DigNum (strict)"("DisabledEnum"=w1790) -> ()  [unwired: 2 in, 2 out]
                n1146 = property on="Frame Transfer 4" class="Bool (strict)"("DisabledEnum"=w1790) -> ()  [unwired: 2 in, 2 out]
                n1147 = property on="Vertical Clock Voltage 4" class="Ring (strict)"("DisabledEnum"=w1790) -> ()  [unwired: 2 in, 2 out]
                n1148 = property on="A/D Channel 4" class="DigNum (strict)"("DisabledEnum"=w1790) -> ()  [unwired: 2 in, 2 out]
                n1149 = property on="Image Initial Line 4" class="DigNum (strict)"("DisabledEnum"=w1790) -> ()  [unwired: 2 in, 2 out]
                n1150 = property on="Image Initial Column 4" class="DigNum (strict)"("DisabledEnum"=w1790) -> ()  [unwired: 2 in, 2 out]
                n1151 = property on="Image Final Line 4" class="DigNum (strict)"("DisabledEnum"=w1790) -> ()  [unwired: 2 in, 2 out]
                n1152 = property on="Shutter Openning Time 4" class="DigNum (strict)"("DisabledEnum"=w1790) -> ()  [unwired: 2 in, 2 out]
                n1153 = property on="Shutter Closing Time 4" class="DigNum (strict)"("DisabledEnum"=w1790) -> ()  [unwired: 2 in, 2 out]
                n1154 = property on="Vertical Binning 4" class="DigNum (strict)"("DisabledEnum"=w1790) -> ()  [unwired: 2 in, 2 out]
                n1155 = property on="Horizontal Binning 4" class="DigNum (strict)"("DisabledEnum"=w1790) -> ()  [unwired: 2 in, 2 out]
                n1156 = property on="Acquisition Mode 4" class="Ring (strict)"("DisabledEnum"=w1790) -> ()  [unwired: 2 in, 2 out]
                n1157 = property on="CCD EM Gain 4" class="DigNum (strict)"("DisabledEnum"=w1790) -> ()  [unwired: 2 in, 2 out]
                n1158 = property on="Shutter Mode 4" class="Ring (strict)"("DisabledEnum"=w1790) -> ()  [unwired: 2 in, 2 out]
                n1159 = property on="Shutter TTL 4" class="Ring (strict)"("DisabledEnum"=w1790) -> ()  [unwired: 2 in, 2 out]
                n1160 = property on="Readout Rate 4" class="Ring (strict)"("DisabledEnum"=w1790) -> ()  [unwired: 2 in, 2 out]
                n1161 = property on="Vertical Shift Speed 4" class="Ring (strict)"("DisabledEnum"=w1790) -> ()  [unwired: 2 in, 2 out]
                n1162 = property on="CCD EM Mode 4" class="Ring (strict)"("DisabledEnum"=w1790) -> ()  [unwired: 2 in, 2 out]
                n1163 = property on="Trigger Mode 4" class="Ring (strict)"("DisabledEnum"=w1790) -> ()  [unwired: 2 in, 2 out]
                n1164 = property on="Read Mode 4" class="Ring (strict)"("DisabledEnum"=w1790) -> ()  [unwired: 2 in, 2 out]
                n1165 = property on="Pre-amplification Gain 4" class="Ring (strict)"("DisabledEnum"=w1790) -> ()  [unwired: 2 in, 2 out]
              }
              frame #19 {
                n1166 = Unbundle By Name(w1956) -> ("object_suffix"=w1955:string, "dflat_suffix"=w1954:string, "sflat_suffix"=w1953:string, "dark_suffix"=w1952:string, "zero_suffix"=w1951:string, "focus_suffix"=w1950:string, "suffixAlertVisible"=w1949:bool)
                n1167 = local write "object suffix"(w1955) -> ()
                n1168 = local write "dflat suffix"(w1954) -> ()
                n1169 = local write "sflat suffix"(w1953) -> ()
                n1170 = local write "dark suffix"(w1952) -> ()
                n1171 = local write "zero suffix"(w1951) -> ()
                n1172 = local write "focus suffix"(w1950) -> ()
                n1173 = property on="suffix alert" class="Str"("Visible"=w1949) -> ()  [unwired: 2 in, 2 out]
                n1174 = case shown="True" w1959 {
                  tunnel: [w1960 w1996] -> w1957
                  tunnel: [w1960 w1980] -> w1958
                  tunnel: w1956 -> [_ w1986]
                  frame False {
                    w1960 = FALSE
                  }
                  frame True {
                    w1966 = TRUE
                    # "Pelo menos 1 canal deve \nestar habilitado"
                    n1175 = local read "Preview Temp."() -> (w1985:dbl)
                    n1176 = Unbundle By Name(w1986) -> ("ChannelA_Status.target  temp"=w1982:i16, "ChannelB_Status.target  temp"=w1984:i16, "ChannelC_Status.target  temp"=w1983:i16, "ChannelD_Status.target  temp"=w1981:i16)
                    n1177 = property on="CCD checked 3" class="Bool (strict)"() -> ("Value"=w1992:bool)  [unwired: 2 in, 2 out]
                    n1178 = local read "CH3 on"() -> (w1976:bool)
                    n1179 = local read "CH1on"() -> (w1978:bool)
                    n1180 = property on="CCD checked 2" class="Bool (strict)"() -> ("Value"=w1995:bool)  [unwired: 2 in, 2 out]
                    n1181 = local read "CH2on"() -> (w1977:bool)
                    n1182 = property on="CCD checked 1" class="Bool (strict)"() -> ("Value"=w1999:bool)  [unwired: 2 in, 2 out]
                    n1183 = property on="CCD checked 4" class="Bool (strict)"() -> ("Value"=w1989:bool)  [unwired: 2 in, 2 out]
                    n1184 = local read "CH4 on"() -> (w1975:bool)
                    n1185 = To Word Integer(number=w1985) -> (16bit integer=w1979:i16)
                    n1186 = Select(t=w1999, s=w1978, f=TRUE) -> (s? t:f=w1997:bool)
                    n1187 = local read "CH3 on"() -> (w1968:bool)
                    n1188 = local read "CH4 on"() -> (w1967:bool)
                    n1189 = Compound Arithmetic op=OR(w1978, w1977, w1976, w1975) -> (w1965:bool)
                    n1190 = local read "CH2on"() -> (w1969:bool)
                    n1191 = Select(t=w1992, s=w1976, f=TRUE) -> (s? t:f=w1990:bool)
                    n1192 = Select(t=w1995, s=w1977, f=TRUE) -> (s? t:f=w1993:bool)
                    n1193 = Select(t=w1989, s=w1975, f=TRUE) -> (s? t:f=w1987:bool)
                    n1194 = Equal?(x=w1979, y=w1984) -> (x = y?=w1973:bool)
                    n1195 = Equal?(x=w1979, y=w1983) -> (x = y?=w1972:bool)
                    n1196 = Equal?(x=w1979, y=w1981) -> (x = y?=w1971:bool)
                    n1197 = Equal?(x=w1979, y=w1982) -> (x = y?=w1974:bool)
                    n1198 = local read "CH1on"() -> (w1970:bool)
                    n1199 = Select(t=w1974, s=w1970, f=w1966) -> (s? t:f=w1964:bool)
                    n1200 = Select(t=w1972, s=w1968, f=w1966) -> (s? t:f=w1962:bool)
                    n1201 = Select(t=w1971, s=w1967, f=w1966) -> (s? t:f=w1961:bool)
                    n1202 = Select(t=w1973, s=w1969, f=w1966) -> (s? t:f=w1963:bool)
                    n1203 = Compound Arithmetic op=AND(w1997, w1993, w1990, w1987, w1965) -> (w1996:bool)
                    n1204 = Compound Arithmetic op=AND(w1965, w1964, w1963, w1962, w1961) -> (w1980:bool)
                  }
                }
                "SET Temp status" <- w1958
                "SET CCD status" <- w1957
              }
            }
            n1205 = In Range and Coerce(upper limit=u32 226, x=w292, lower limit=u32 220 ("upper limit")) -> (In Range?=w331:bool)  [unwired: 1 out]
            n1206 = call-dynamic "Read TelFocus.lvclass.vi"("error in (no error)"=w313, "S4GUI in"=w314) -> ("error out"=w311:errorcluster, "TelFocus.lvclass"=w312:refnum<class "TelFocus.lvclass">)  [unwired: 7 in, 1 out]
            n1207 = Select(t="STOP", s=w331, f="INIT") -> (s? t:f=w330:string)
            n1208 = call-dynamic "Read focus #stepsdone.vi"("error in (no error)"=w311, "TelFocus in"=w312) -> ("focus #stepsdone"=→"steps done":u32)  [unwired: 7 in, 2 out]
            n1209 = property on="Init mode" class="Bool"(error in=w313, "Blinking"=w331, "Caption.Visible"=w331, "BoolText.Text"=w330) -> (error out=w332:errorcluster)  [unwired: 1 in, 1 out]
            n1210 = call-dynamic "Read cyclesDone.vi"("error in (no error)"=w332, "S4GUI in"=w314) -> ("error out"=w324:errorcluster, "cyclesDone"=w316:u32, "S4GUI out"=w326:refnum<class "S4GUI.lvclass">)  [unwired: 7 in]
            "#Cycles Done" <- w316
            n1211 = call-dynamic "Read cycles wprot.vi"("error in (no error)"=w324, "S4GUI in"=w326) -> ("cycles wprot"=→"Cycles Counter":u32)  [unwired: 7 in, 2 out]
            n1212 = Number To Decimal String(number=w316) -> (decimal integer string=w317:string)  [unwired: 1 in]
            n1213 = Concatenate Strings("#Cycles Done ", w317) -> (w315:string)
            n1214 = property on="#Cycles Done" class="Slide (strict)"("Caption.Text"=w315) -> ()  [unwired: 2 in, 2 out]
            n1215 = call "Read Instrument.lvclass.vi"("error in (no error)"=w324, "S4ACS_GUI in"=w326) -> ("error out"=w340:errorcluster, "Instrument.lvclass"=w338:refnum<class "Instrument.lvclass">, "S4ACS_GUI out"=w341:refnum<class "S4GUI.lvclass">)  [unwired: 7 in]
            n1216 = call-dynamic "Write mode.vi"("error in (no error)"=w340, "mode"=w327, "Instrument in"=w338) -> ("error out"=w339:errorcluster, "Instrument out"=w337:refnum<class "Instrument.lvclass">)  [unwired: 7 in]
            n1217 = call "Write Instrument.lvclass.vi"("error in (no error)"=w339, "Instrument.lvclass"=w337, "S4ACS_GUI in"=w341) -> ("error out"=w322:errorcluster, "S4ACS_GUI out"=w323:refnum<class "S4GUI.lvclass">)  [unwired: 7 in]
            n1218 = call-dynamic "Read Error Msg.vi"("error in (no error)"=w322, "S4GUI in"=w323) -> ("error out"=w319:errorcluster, "Error Msg"=w301:string, "S4GUI out"=w306:refnum<class "S4GUI.lvclass">)  [unwired: 7 in]
            "Last Error" <- w301
            n1219 = Match Pattern(string=w301, regular expression=w320) -> (match substring=w321:string)  [unwired: 1 in, 3 out]
            n1220 = Equal?(x=w321, y=w320) -> (x = y?=w300:bool)
            n1221 = Match Pattern(string=w301, regular expression=w302) -> (match substring=w303:string)  [unwired: 1 in, 3 out]
            n1222 = Equal?(x=w303, y=w302) -> (x = y?=w299:bool)
            n1223 = Or(x=w300, y=w299) -> (x .or. y?=w298:bool)
            n1224 = property on="Last Error" class="Str"(error in=w319, "Blinking"=w298) -> (error out=w304:errorcluster)  [unwired: 1 in, 1 out]
